vi "Version Manager.vi"(8 "error in (no error)":errorcluster, 11 "Device Item Ref In in":T1 format="%.0x") -> (0 "error out":errorcluster, 3 "Device Item Ref In out":T1 format="%.0x")   [LabVIEW 2018, in "NI-XNET Monitor System Explorer.lvlib"]
uses:
  NI-XNET Monitor System Explorer.lvlib
  <vilib>/NI Veristand/Custom Device API/Custom Device Item Ref.ctl
  Shared/Constants.vi
  <vilib>/NI Veristand/Custom Device API/Custom Device API.lvlib
  Shared/NI-XNET Monitor Shared.lvlib
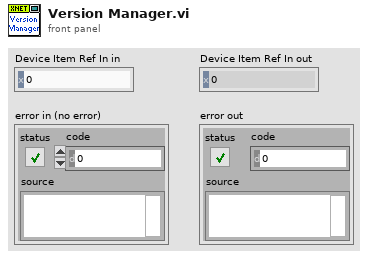
[diagram p1: front panel]
types:
  T1 = typedef "Custom Device API.lvlib/Custom Device Item Ref.ctl" = u64
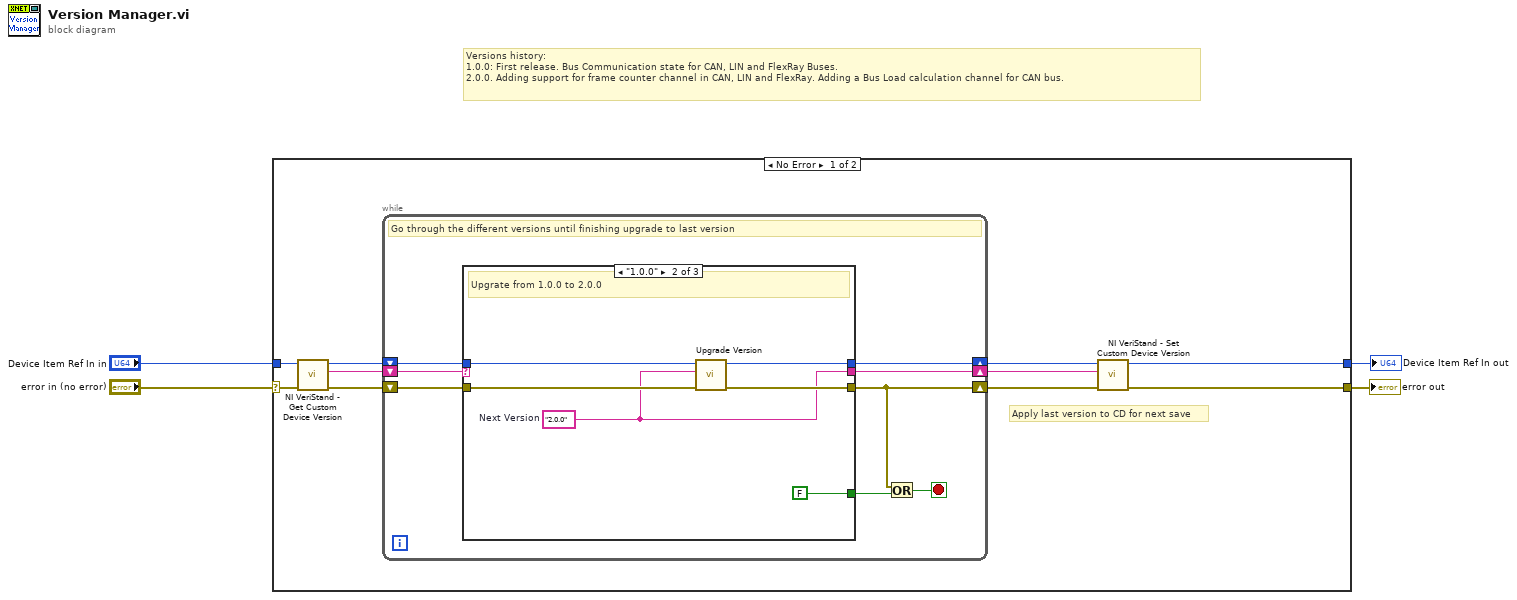
[diagram p0: block diagram]
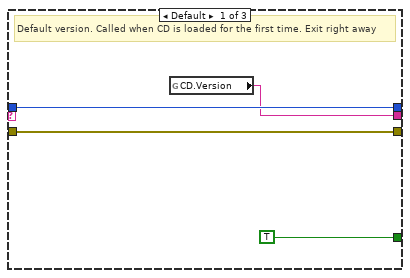
[diagram p2: hidden frame]
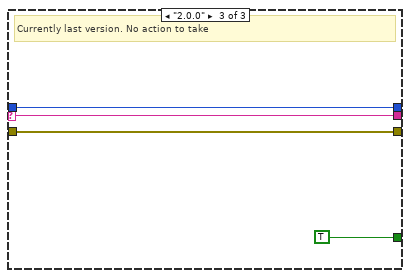
[diagram p3: hidden frame]
diagram:
  # "Versions history:\n1.0.0: First release. Bus Communication state for CAN, LIN and FlexRay Buses.\n2.0.0. Adding support for frame counter channel in CAN, LIN and FlexRay. Adding a Bus Load calculation channel for CAN bus."
  n1 = case shown="No Error" "error in (no error)" {
    selector: "error in (no error)" -> [w13 w37]
    tunnel: "Device Item Ref In in" -> [w14 w38]
    tunnel: [w12 w38] -> w2
    tunnel: [w11 w37] -> w1
    frame No Error {
      # "Apply last version to CD for next save"
      n2 = call <vilib>:"NI VeriStand - Get Custom Device Version.vi"("error in (no error)"=w13, "Device Ref in"=w14) -> ("error out"=w9:errorcluster, "Value"=w5:string, "Device Ref out"=w10:T1)  [unwired: 7 in]
      n3 = while {
        shift-right: [w16] -> w7
        shift-left: w9 -> [w20]
        shift-right: [w17] -> w8
        shift-left: w10 -> [w21]
        shift-right: [w15] -> w6
        shift-left: w5 -> [w22]
        stop <- w19 stop-if-true
        # "Go through the different versions until finishing upgrade to last version"
        n4 = case shown="\"1.0.0\"" w22 {
          selector: w22 -> [_ _ w33]
          tunnel: w21 -> [w25 w30 w35]
          tunnel: w20 -> [w24 w31 w34]
          tunnel: [TRUE FALSE TRUE] -> w18
          tunnel: [w25 w29 w35] -> w17
          tunnel: [w24 w28 w34] -> w16
          tunnel: [w23 w27 w33] -> w15
          frame Default {
            # "Default version. Called when CD is loaded for the first time. Exit right away"
            n5 = global read "Constants.vi" "CD.Version"() -> (w23:string)
          }
          frame "1.0.0" {
            w27 = "2.0.0"  # Next Version
            # "Upgrate from 1.0.0 to 2.0.0"
            n6 = call "Upgrade Version.vi"("error in (no error)"=w31, "New Version"=w27, "Device Item Ref In in"=w30) -> ("error out"=w28:errorcluster, "Device Item Ref In out"=w29:T1)  [unwired: 7 in]
          }
          frame "2.0.0" {
            # "Currently last version. No action to take"
          }
        }
        n7 = Or(x=w16, y=w18) -> (x .or. y?=w19:bool)
      }
      n8 = call <vilib>:"NI VeriStand - Set Custom Device Version.vi"("error in (no error)"=w7, "Value"=w6, "Device Ref in"=w8) -> ("error out"=w11:errorcluster, "Device Ref out"=w12:T1)  [unwired: 7 in]
    }
    frame Error {
    }
  }
  "error out" <- w1
  "Device Item Ref In out" <- w2
